vi "Find Contours.vi"(0 "Image Src":T1, 1 "Background Image":T1, 2 "Median Filter Size":i32=5 min=0 max=7, 3 "Range":cluster{"Lower value":sgl, "Upper value":sgl}={"Lower value"=3000.0, "Upper value"=32768.0} {"Upper value" format="%.2f"; "Lower value" format="%.2f"}, 4 "Curve Parameters":T3={"Extraction Mode"=1, "Edge Threshold"=75, "Edge Filter Size"=0, "Min Length"=25, "Row Search Step Size"=15, "Col Search Step Size"=15, "Max Endpoint Gap"=10, "Closed"=TRUE, "Subpixel"=TRUE} {"Extraction Mode" items=["Normal", "Uniform Regions"]; "Edge Filter Size" items=["Fine", "Normal", "Contour Tracing"]; "Max Endpoint Gap" min=0; "Col Search Step Size" min=1 max=255 step=1; "Row Search Step Size" min=1 max=255 step=1; "Min Length" min=0; "Edge Threshold" min=1 max=350 step=1}, 5 "error in (no error)":errorcluster) -> (14 "Image Src Dup":T1, 15 "Background Subtracted Image":T1, 17 "Curves":T2[](array[typedef]) {"Points"."Y" format="%.2f"; "Points"."X" format="%.2f"}, 19 "error out":errorcluster)   [LabVIEW 2011]
uses:
  <vilib>/vision/Pattern Matching.llb/IMAQ Curve Parameters.ctl
  <vilib>/vision/Analysis.llb/IMAQ ExtractCurvesCurve.ctl
  <vilib>/vision/Image Controls.llb/IMAQ Image.ctl
  <vilib>/vision/NI_Vision_Development_Module.lvlib
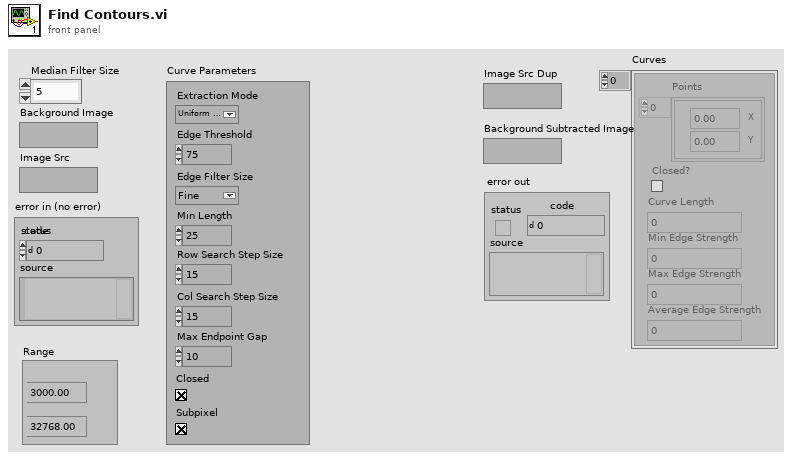
[diagram p1: front panel]
types:
  T1 = typedef "IMAQ Image.ctl" = refnum<image>
  T2 = typedef "IMAQ ExtractCurvesCurve.ctl" = cluster{"Points":cluster{"X":dbl, "Y":dbl}[], "Closed?":bool, "Curve Length":dbl, "Min Edge Strength":dbl, "Max Edge Strength":dbl, "Average Edge Strength":dbl}
  T3 = typedef "IMAQ Curve Parameters.ctl" = cluster{"Extraction Mode":u32, "Edge Threshold":i32, "Edge Filter Size":u32, "Min Length":i32, "Row Search Step Size":i32, "Col Search Step Size":i32, "Max Endpoint Gap":i32, "Closed":bool, "Subpixel":bool}
  T4 = typedef "Image Type" = u32
  T5 = cluster{"Median Filter Size":i32, "Median Filter Size":i32, i32}
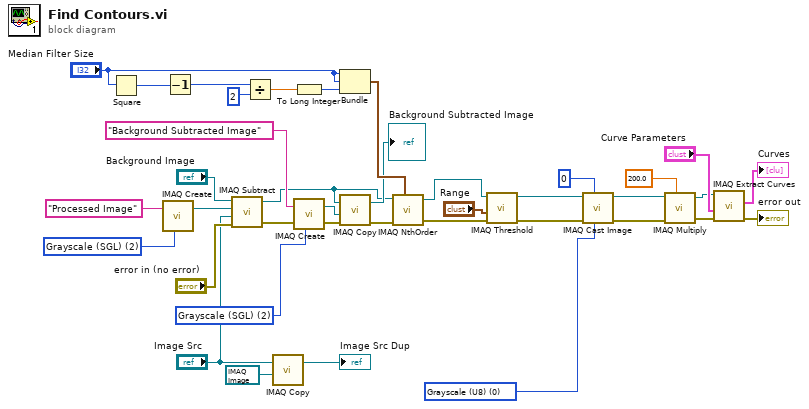
[diagram p0: block diagram]
diagram:
  w13 = T4 2 items=["Grayscale (U8)", "Grayscale (I16)", "Grayscale (SGL)", "Complex (CSG)", "RGB (U32)", "HSL (U32)", "RGB (U64)", "Grayscale (U16)"] ("Image Type")
  w16 = T4 0 items=["Grayscale (U8)", "Grayscale (I16)", "Grayscale (SGL)", "Complex (CSG)", "RGB (U32)", "HSL (U32)", "RGB (U64)", "Grayscale (U16)"] ("Image Type")
  w27 = T4 2 items=["Grayscale (U8)", "Grayscale (I16)", "Grayscale (SGL)", "Complex (CSG)", "RGB (U32)", "HSL (U32)", "RGB (U64)", "Grayscale (U16)"] ("Image Type")
  n1 = Square(x="Median Filter Size") -> (x^2=w36:i32)
  n2 = call "IMAQ Create"("Image Name"="Processed Image", "Image Type"=w27) -> ("New Image"=w19:T1)  [unwired: 3 in, 1 out]
  n3 = Decrement(x=w36) -> (x-1=w35:i32)
  n4 = call "IMAQ Subtract"("Image Src A"="Background Image", "Image Dst"=w19, "Image Src B"="Image Src", "error in (no error)"="error in (no error)") -> ("Image Dst Out"=w3:T1, "error out"=w2:errorcluster)  [unwired: 3 in]
  n5 = Divide(x=w35, y=2) -> (x/y=w33:dbl)
  n6 = call "IMAQ Copy"("Image Dst"=T1 refnum, "Image Src"="Image Src") -> ("Image Dst Out"=→"Image Src Dup":T1)  [unwired: 4 in, 1 out]
  n7 = To Long Integer(number=w33) -> (32bit integer=w32:i32)
  n8 = call "IMAQ Create"("Image Name"="Background Subtracted Image", "Image Type"=w13, "error in (no error)"=w2) -> ("New Image"=w11:T1, "error out"=w12:errorcluster)  [unwired: 2 in]
  n9 = Bundle("Median Filter Size"="Median Filter Size", "Median Filter Size"="Median Filter Size", w32) -> (w29:T5)  [unwired: 1 in]
  n10 = call "IMAQ Copy"("error in (no error)"=w12, "Image Dst"=w11, "Image Src"=w3) -> ("error out"=w1:errorcluster, "Image Dst Out"=→"Background Subtracted Image":T1)  [unwired: 3 in]
  n11 = call "IMAQ NthOrder"("Image Src"=w3, "Size & Order #"=w29, "error in (no error)"=w1) -> ("Image Dst Out"=w10:T1, "error out"=w23:errorcluster)  [unwired: 4 in]
  n12 = call "IMAQ Threshold"("error in (no error)"=w23, "Range"="Range", "Image Src"=w10) -> ("error out"=w18:errorcluster, "Image Dst Out"=w17:T1)  [unwired: 7 in]
  n13 = call "IMAQ Cast Image"("Image Type"=w16, "# Shifts"=0, "error in (no error)"=w18, "Image Src"=w17) -> ("error out"=w8:errorcluster, "Image Dst Out"=w5:T1)  [unwired: 6 in]
  n14 = call "IMAQ Multiply"("Image Src A"=w5, "Constant"=sgl 200.0, "error in (no error)"=w8) -> ("Image Dst Out"=w6:T1, "error out"=w7:errorcluster)  [unwired: 4 in]
  n15 = call "IMAQ Extract Curves"("error in (no error)"=w7, "Curve Parameters"="Curve Parameters", "Image"=w6) -> ("error out"=→"error out":errorcluster, "Curves"=→"Curves":T2[])  [unwired: 6 in, 1 out]
